vi "reference.vi"(2 "set?":bool, 4 "coordinates (pixel)":refnum<vi>, 5 "Pickcoord. (pixel)":refnum<vi>) -> (0 "coordinates (pixel) 2":refnum<vi>, 1 "Pickcoord. (pixel) 2":refnum<vi>)   [LabVIEW 2009]
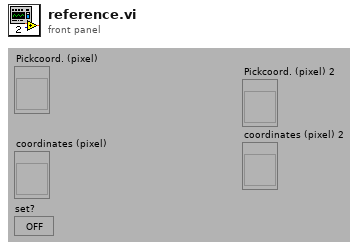
[diagram p1: front panel]
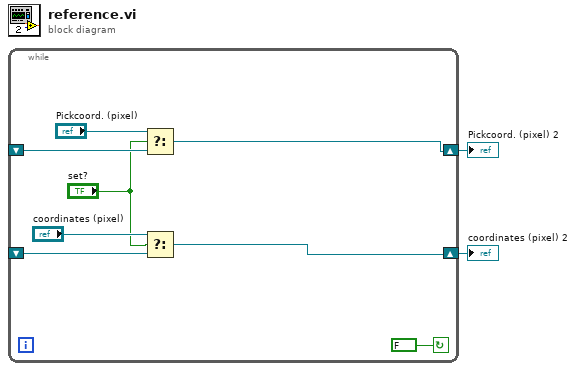
[diagram p0: block diagram]
diagram:
  n1 = while {
    shift-right: [w6] -> w2
    shift-left: _ -> [w5]
    shift-right: [w7] -> w1
    shift-left: _ -> [w8]
    stop <- FALSE continue-if-true
    n2 = Select(t="Pickcoord. (pixel)", s="set?", f=w5) -> (s? t:f=w6:refnum<vi>)
    n3 = Select(t="coordinates (pixel)", s="set?", f=w8) -> (s? t:f=w7:refnum<vi>)
  }
  "Pickcoord. (pixel) 2" <- w2
  "coordinates (pixel) 2" <- w1
